vi "Run Server.vi"() -> ()   [LabVIEW 2021, in "CIFCoreChannel_server.lvlib"]
uses:
  CIFCoreChannel_server.lvlib
  <vilib>/gRPC/LabVIEW gRPC Servicer/ServiceBase/ServiceBase.lvclass
  <vilib>/gRPC/LabVIEW gRPC Servicer/Servicer/Servicer.lvclass
panel:
  in  "Async [T] / Sync [F]":bool
  out "Listening Port":i32
  in  "Stop":bool
  in  "Server Address":string="localhost:50051"
  in  "Server Certificate File (.crt)":path
  in  "Server Key File (.key)":path
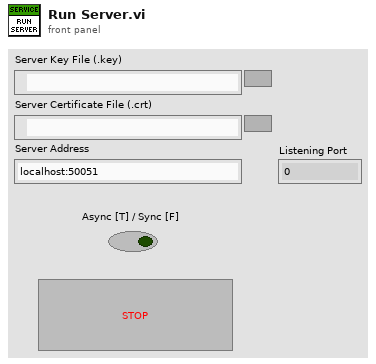
[diagram p1: front panel]
types:
  T1 = enum32{"Invalid", "Standard", "Closed", "Hidden", "Minimized", "Maximized"}
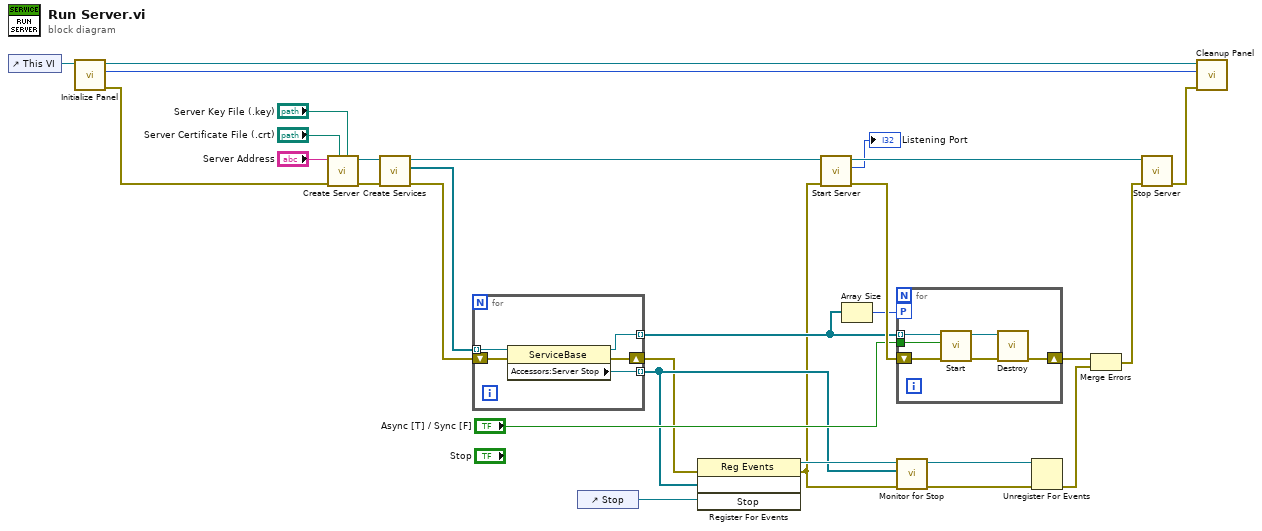
[diagram p0: block diagram]
diagram:
  n1 = control-ref of="This VI"() -> (w7:refnum<vi>)
  n2 = call "Initialize Panel.vi"("vi reference in"=w7) -> ("error out"=w8:errorcluster, "initial window state"=w5:T1, "vi reference out"=w6:refnum<vi>)  [unwired: 8 in]
  n3 = call <vilib>:"Create Server.vi"("Server Key File (.key)"="Server Key File (.key)", "Server Certificate File (.crt)"="Server Certificate File (.crt)", "error in"=w8, "Server Address"="Server Address") -> ("error out"=w3:errorcluster, "gRPC server out"=w23:refnum<class "Servicer.lvclass">)  [unwired: 6 in]
  n4 = call "Create Services.vi"("error in (no error)"=w3, "gRPC server in"=w23) -> ("error out"=w2:errorcluster, "gRPC services out"=w1:refnum<class "ServiceBase.lvclass">[], "gRPC server out"=w22:refnum<class "Servicer.lvclass">)  [unwired: 7 in]
  n5 = for {
    tunnel: [w33] -> w17 mode=indexing
    shift-right: [w32] -> w16
    shift-left: w2 -> [w30]
    tunnel: [w34] -> w18 mode=indexing
    tunnel: w1 -> [w31] mode=indexing
    n6 = property class="ServiceBase"(reference=w31, error in=w30) -> (reference out=w34:refnum<class "ServiceBase.lvclass">, error out=w32:errorcluster, "Accessors:Server Stop"=w33:refnum<user-event>)
  }
  n7 = control-ref of="Stop"() -> (w12:refnum<vi>)
  n8 = register-events(error in=w16, w17, w12) -> (reference out=w25:refnum<event-registration>, error out=w15:errorcluster)  [unwired: 1 in]
  n9 = call <vilib>:"Start Server.vi"("error in"=w15, "gRPC server in"=w22) -> ("error out"=w21:errorcluster, "Listening Port"=→"Listening Port":i32, "gRPC server out"=w29:refnum<class "Servicer.lvclass">)  [unwired: 7 in]
  n10 = Array Size(array=w18) -> (size(s)=w19:i32)
  n11 = for {
    tunnel: w18 -> [w38] mode=indexing
    tunnel: "Async [T] / Sync [F]" -> [w36]
    workers-P: w19 -> [_]
    shift-right: [w35] -> w14
    shift-left: w21 -> [w37]
    n12 = call-dynamic "Start.vi"("error in"=w37, "ASync [T]"=w36, "gRPC service in"=w38) -> ("error out"=w39:errorcluster, "gRPC service out"=w40:refnum<class "ServiceBase.lvclass">)  [unwired: 7 in]
    n13 = call-dynamic "Destroy.vi"("error in"=w39, "gRPC service in"=w40) -> ("error out"=w35:errorcluster)  [unwired: 8 in, 1 out]
  }
  n14 = call "Monitor for Stop.vi"("error in (no error)"=w15, "service stop events"=w17, "Event Registration Refnum in"=w25) -> ("error out"=w9:errorcluster, "Event Registration Refnum out"=w11:refnum<event-registration>)  [unwired: 7 in]
  n15 = Unregister For Events(event registration refnum=w11, error in=w9) -> (error out=w10:errorcluster)
  n16 = Merge Errors(w14, w10) -> (w13:errorcluster)
  n17 = call <vilib>:"Stop Server.vi"("error in"=w13, "gRPC server in"=w29) -> ("error out"=w4:errorcluster)  [unwired: 9 in]
  n18 = call "Cleanup Panel.vi"("error in (no error)"=w4, "initial window state"=w5, "vi reference in"=w6) -> ()  [unwired: 7 in, 2 out]
